vi "Get Cell Values (VAR).vi"(7 "Sheet Name in":string, 8 "error in":errorcluster, 10 "Cell Range":string="A1:B1", 11 "SpreadsheetDoc in":refnum<k24>) -> (0 "error out":errorcluster, 2 "Cell Values":variant[][](array[variant]), 3 "SpreadsheetDoc out":refnum<k24>)   [LabVIEW 2019, in "Open Xml.lvlib"]
uses:
  Open Xml.lvlib
  D:/git/Open-Xml-LabVIEW/Source/DocumentFormat.OpenXml.dll
  DocumentFormat.OpenXml.dll
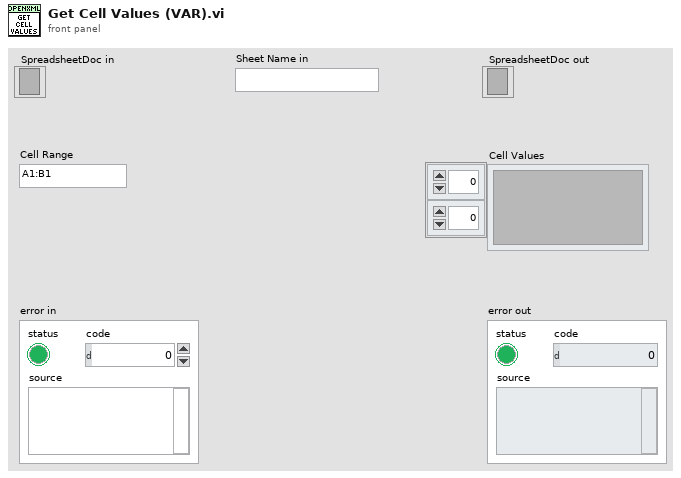
[diagram p1: front panel]
types:
  T1 = typedef "Open Xml.lvlib/Cell DataType.ctl" = enum16{"Void", "Boolean", "Number", "Error", "SharedString", "String", "InlineString", "Date"}
  T2 = cluster{"Number":dbl, "String":string, "Boolean":bool, "Time Stamp":timestamp, "Error":errorcluster}
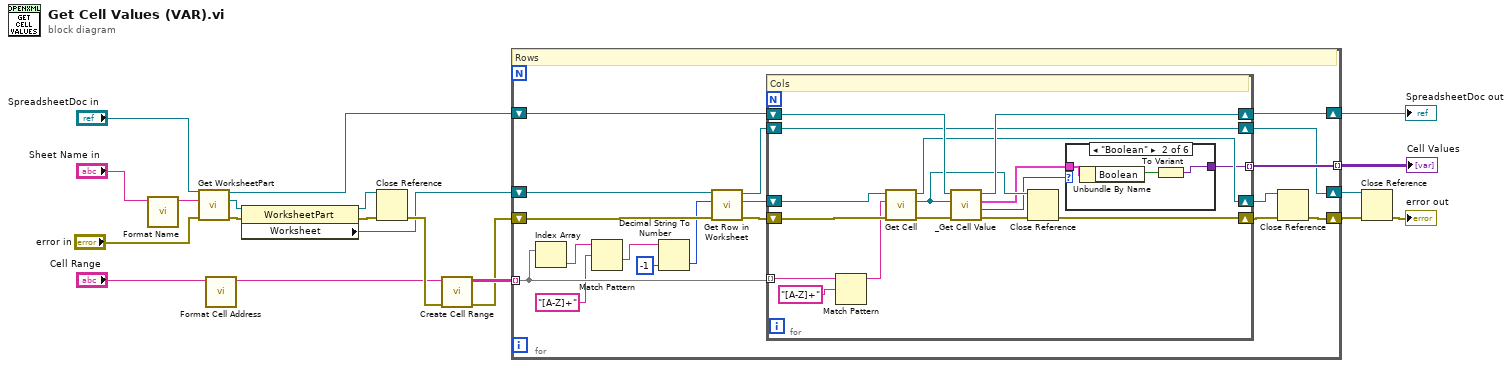
[diagram p0: block diagram]
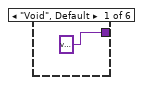
[diagram p2: hidden frame]
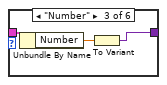
[diagram p3: hidden frame]
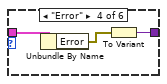
[diagram p4: hidden frame]
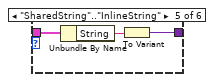
[diagram p5: hidden frame]
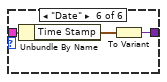
[diagram p6: hidden frame]
diagram:
  n1 = call "Format Name.vi"("Sheet Name"="Sheet Name in") -> ("Formatted Sheet Name"=w1:string)  [unwired: 10 in]
  n2 = call "Get WorksheetPart.vi"("error in"="error in", "Sheet Name"=w1, "SpreadsheetDoc in"="SpreadsheetDoc in") -> ("error out"=w9:errorcluster, "WorksheetPart"=w8:refnum<k24>, "SpreadsheetDoc out"=w15:refnum<k24>)  [unwired: 5 in, 1 out]
  n3 = call "Format Cell Address.vi"("Cell Address"="Cell Range") -> ("Formatted Cell Address"=w2:string)  [unwired: 10 in]
  n4 = property class="WorksheetPart"(reference=w8, error in=w9) -> (reference out=w5:refnum<k24>, error out=w7:errorcluster, "Worksheet"=w4:refnum<k24>)
  n5 = Close Reference(reference=w5, error in (no error)=w7) -> (error out=w6:errorcluster)
  n6 = call "Create Cell Range.vi"("error in"=w6, "Cell Range"=w2) -> ("error out"=w12:errorcluster, "Cell Range"=w18:string[][])  [unwired: 8 in]
  n7 = for {
    tunnel: w18 -> [w29] mode=indexing
    tunnel: [w35] -> w14 mode=indexing
    shift-right: [w37] -> w19
    shift-left: w15 -> [w36]
    shift-right: [w22] -> w20
    shift-left: w12 -> [w33]
    shift-right: [w34] -> w13
    shift-left: w4 -> [w31]
    # "Rows"
    n8 = Index Array(array=w29) -> (element=w28:string)  [unwired: 1 in]
    n9 = Match Pattern(string=w28, regular expression="[A-Z]+") -> (after substring=w25:string)  [unwired: 1 in, 3 out]
    n10 = Decimal String To Number(string=w25, default (0L)=-1 ("default (0 I32)")) -> (number=w24:i32)  [unwired: 1 in, 1 out]
    n11 = call "Get Row in Worksheet.vi"("error in"=w33, "RowIndex"=w24, "Worksheet in"=w31) -> ("error out"=w32:errorcluster, "Row out"=w23:refnum<k24>, "Worksheet out"=w30:refnum<k24>)  [unwired: 6 in]
    n12 = for {
      tunnel: [w40] -> w35 mode=indexing
      shift-right: [w39] -> w38
      shift-left: w32 -> [w53]
      shift-right: [w51] -> w37
      shift-left: w36 -> [w52]
      tunnel: w29 -> [w46] mode=indexing
      shift-right: [w43] -> w21
      shift-left: w23 -> [w44]
      shift-right: [w45] -> w34
      shift-left: w30 -> [w45]
      # "Cols"
      n13 = Match Pattern(string=w46, regular expression="[A-Z]+") -> ()  [unwired: 1 in, 4 out]
      n14 = call "Get Cell.vi"("error in"=w53, "Cell Address"=w46, "Row in"=w44) -> ("error out"=w50:errorcluster, "Cell"=w48:refnum<k24>, "Row out"=w43:refnum<k24>)  [unwired: 6 in]
      n15 = call "_Get Cell Value.vi"("error in"=w50, "Cell"=w48, "SpreadsheetDoc in"=w52) -> ("error out"=w49:errorcluster, "Type"=w42:T1, "Cell Value"=w41:T2, "SpreadsheetDocument out"=w51:refnum<k24>)  [unwired: 5 in]
      n16 = Close Reference(reference=w48, error in (no error)=w49) -> (error out=w39:errorcluster)
      n17 = case shown="\"Boolean\"" w42 {
        tunnel: w41 -> [_ w57 w60 w63 w66 w69]
        tunnel: [variant w55 w58 w61 w64 w68] -> w40
        frame "Void", Default {
        }
        frame "Boolean" {
          n18 = Unbundle By Name(w57) -> ("Boolean"=w56:bool)
          n19 = To Variant(anything=w56) -> (Variant=w55:variant)
        }
        frame "Number" {
          n20 = Unbundle By Name(w60) -> ("Number"=w59:dbl)
          n21 = To Variant(anything=w59) -> (Variant=w58:variant)
        }
        frame "Error" {
          n22 = Unbundle By Name(w63) -> ("Error"=w62:errorcluster)
          n23 = To Variant(anything=w62) -> (Variant=w61:variant)
        }
        frame "SharedString".."InlineString" {
          n24 = Unbundle By Name(w66) -> ("String"=w65:string)
          n25 = To Variant(anything=w65) -> (Variant=w64:variant)
        }
        frame "Date" {
          n26 = Unbundle By Name(w69) -> ("Time Stamp"=w67:timestamp)
          n27 = To Variant(anything=w67) -> (Variant=w68:variant)
        }
      }
    }
    n28 = Close Reference(reference=w21, error in (no error)=w38) -> (error out=w22:errorcluster)
  }
  "SpreadsheetDoc out" <- w19
  "Cell Values" <- w14
  n29 = Close Reference(reference=w13, error in (no error)=w20) -> (error out=→"error out":errorcluster)
